vi "Check Firmware Version.vi"(8 "Error In":errorcluster, 11 "LINX Device Config":T1) -> (0 "Error Out":errorcluster, 3 "LINX Device Config":T1)   [LabVIEW 2020, in "LMH-LINX.lvlib" / "Device.lvlib"]
uses:
  Device.lvlib
  Type Defs/LINX Device Config.ctl
  Type Defs/Interface.ctl
  Type Defs/TCP Config.ctl
  Type Defs/Channels.ctl
  Type Defs/Error Type.ctl
  LMH-LINX.lvlib
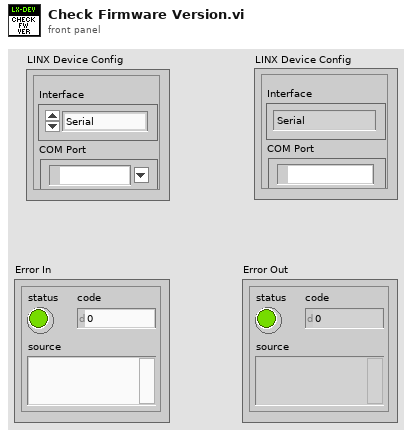
[diagram p1: front panel]
types:
  T1 = typedef "LMH-LINX.lvlib/Device.lvlib/LINX Device Config.ctl" = cluster{"Interface":T2, "COM Port":refnum<visa-resource-name>, "TCP Configuration":T3, "Device Family":u8, "Device ID":u8, "Device Name":string, "TCP Ref":refnum<k5>, "Channels":T4}
  T2 = typedef "LMH-LINX.lvlib/Interface.ctl" = enum16{"Serial", "TCP"}
  T3 = typedef "LMH-LINX.lvlib/Device.lvlib/TCP Config.ctl" = cluster{"IP Address":string, "Port":u16}
  T4 = typedef "LMH-LINX.lvlib/Channels.ctl" = cluster{"DI":u8[], "DO":u8[], "AI":u8[], "AO":u8[], "PWM":u8[], "QE":u8[], "UART":u8[], "I2C 2":u8[], "SPI":u8[], "CAN":u8[], "Servo":u8[], "AI Ref (V)":dbl, "AI Resolution (Bits)":u8, "AO Ref (V)":dbl, "AO Resolution (Bits)":u8}
  T5 = typedef "LMH-LINX.lvlib/Error Type.ctl" = enum16{"Unknown", "Timeout", "Corrupt Return Packet", "Unable To Connect", "Command Not Supported", "Channel DNE", "Invalid COM Config", "Firmware Version Mismatch", "myRIO Support", "CMD Specific Error", "Local IO Not Supported"}
  T6 = typedef "LMH-LINX.lvlib/Device.lvlib/Firmware Version.ctl" = cluster{"Major":u8, "Minor":u8, "SubMinor":u8}
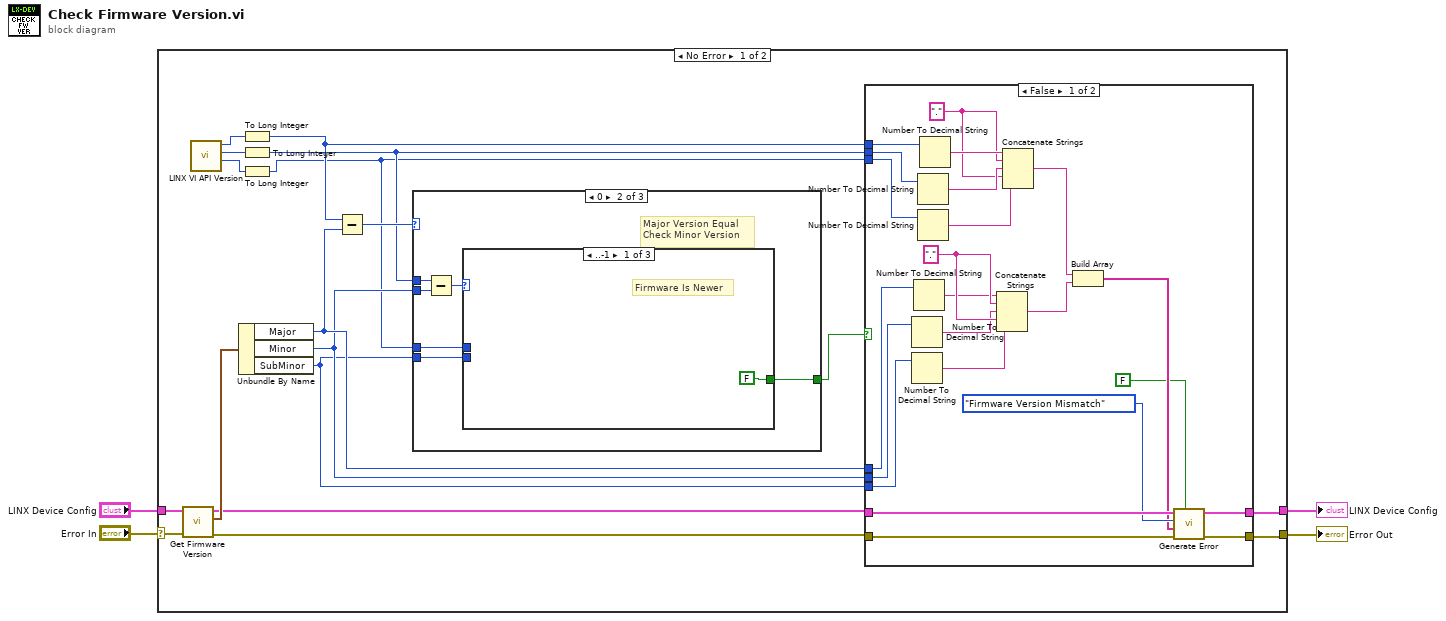
[diagram p0: block diagram]
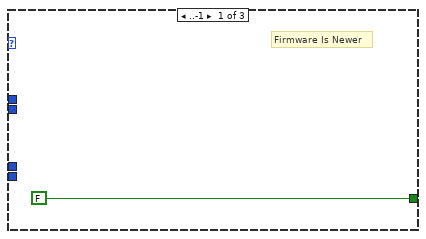
[diagram p2: hidden frame]
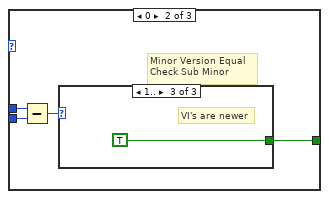
[diagram p3: hidden frame]
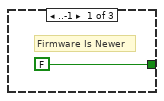
[diagram p4: hidden frame]
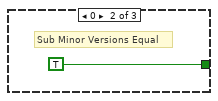
[diagram p5: hidden frame]
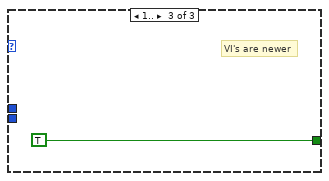
[diagram p6: hidden frame]
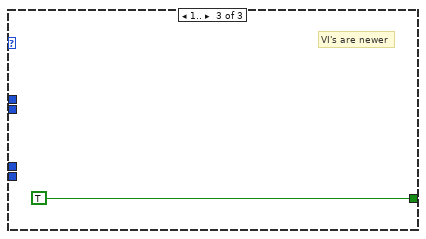
[diagram p7: hidden frame]
diagram:
  n1 = case shown="No Error" "Error In" {
    selector: "Error In" -> [w16 w65]
    tunnel: "LINX Device Config" -> [w22 w66]
    tunnel: [w18 w66] -> w3
    tunnel: [w17 w65] -> w2
    frame No Error {
      n2 = call "Get Firmware Version.vi"("Error In"=w16, "LINX Device Config"=w22) -> ("Error Out"=w19:errorcluster, "LINX Firmware Version"=w21:T6, "LINX Device Config"=w20:T1)  [unwired: 7 in]
      n3 = call "LINX VI API Version.vi"() -> ("SubMinor"=w6:u8, "Minor"=w8:u8, "Major"=w10:u8)  [unwired: 9 in]
      n4 = Unbundle By Name(w21) -> ("Major"=w14:u8, "Minor"=w13:u8, "SubMinor"=w12:u8)
      n5 = To Long Integer(number=w10) -> (32bit integer=w9:i32)
      n6 = To Long Integer(number=w8) -> (32bit integer=w7:i32)
      n7 = To Long Integer(number=w6) -> (32bit integer=w5:i32)
      n8 = Subtract(x=w9, y=w14) -> (x-y=w15:i32)
      n9 = case shown="0" w15 {
        tunnel: [FALSE w26 TRUE] -> w11
        tunnel: w7 -> [_ w29 _]
        tunnel: w13 -> [_ w28 _]
        tunnel: w5 -> [_ w25 _]
        tunnel: w12 -> [_ w24 _]
        frame ..-1 {
          # "Firmware Is Newer"
        }
        frame 0 {
          # "Major Version Equal\nCheck Minor Version"
          n10 = Subtract(x=w29, y=w28) -> (x-y=w27:i32)
          n11 = case shown="..-1" w27 {
            tunnel: [FALSE w31 TRUE] -> w26
            tunnel: w25 -> [_ w34 _]
            tunnel: w24 -> [_ w33 _]
            frame ..-1 {
              # "Firmware Is Newer"
            }
            frame 0 {
              # "Minor Version Equal\nCheck Sub Minor"
              n12 = Subtract(x=w34, y=w33) -> (x-y=w32:i32)
              n13 = case shown="1.." w32 {
                tunnel: [FALSE TRUE TRUE] -> w31
                frame ..-1 {
                  # "Firmware Is Newer"
                }
                frame 0 {
                  # "Sub Minor Versions Equal"
                }
                frame 1.. {
                  # "VI's are newer"
                }
              }
            }
            frame 1.. {
              # "VI's are newer"
            }
          }
        }
        frame 1.. {
          # "VI's are newer"
        }
      }
      n14 = case shown="False" w11 {
        tunnel: w9 -> [w62 _]
        tunnel: w7 -> [w61 _]
        tunnel: w5 -> [w60 _]
        tunnel: w14 -> [w49 _]
        tunnel: w13 -> [w48 _]
        tunnel: w12 -> [w47 _]
        tunnel: w20 -> [w46 w64]
        tunnel: w19 -> [w45 w63]
        tunnel: [w42 w64] -> w18
        tunnel: [w41 w63] -> w17
        frame False {
          w54 = "." ("string")
          w57 = "." ("string")
          n15 = Number To Decimal String(number=w48) -> (decimal integer string=w53:string)  [unwired: 1 in]
          n16 = Number To Decimal String(number=w47) -> (decimal integer string=w55:string)  [unwired: 1 in]
          n17 = Number To Decimal String(number=w49) -> (decimal integer string=w52:string)  [unwired: 1 in]
          n18 = Number To Decimal String(number=w61) -> (decimal integer string=w58:string)  [unwired: 1 in]
          n19 = Number To Decimal String(number=w60) -> (decimal integer string=w56:string)  [unwired: 1 in]
          n20 = Number To Decimal String(number=w62) -> (decimal integer string=w59:string)  [unwired: 1 in]
          n21 = Concatenate Strings(w52, w54, w53, w54, w55) -> (w51:string)
          n22 = Concatenate Strings(w59, w57, w58, w57, w56) -> (w50:string)
          n23 = Build Array(w50, w51) -> (w43:string[])
          n24 = call "Generate Error.vi"("Is Warning? (False)"=FALSE, "Error In"=w45, "Arguments"=w43, "Error Type"=Error_Type."Firmware Version Mismatch", "LINX Device Config"=w46) -> ("Error Out"=w41:errorcluster, "Dup LINX Device Config"=w42:T1)  [unwired: 5 in]
        }
        frame True {
          # "Firmware Match.  Continue"
        }
      }
    }
    frame Error {
    }
  }
  "Error Out" <- w2
  "LINX Device Config" <- w3
